vi "子vi调用.vi"() -> ()   [LabVIEW 2018]
panel:
  in  "布尔":bool
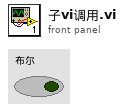
[diagram p1: front panel]
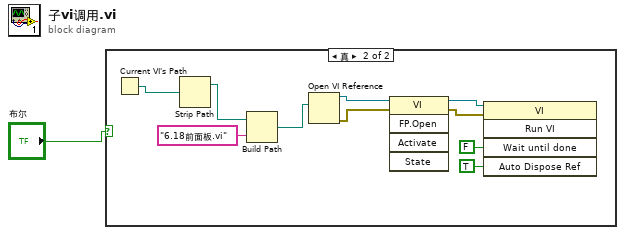
[diagram p0: block diagram]
diagram:
  n1 = case shown="真" "布尔" {
    frame False {
    }
    frame True {
      n2 = Current VI's Path() -> (path=w11:path)
      n3 = Strip Path(path=w11) -> (stripped path=w10:path)  [unwired: 1 out]
      n4 = Build Path(base path=w10, name or relative path="6.18前面板.vi" ("名称或相对路径")) -> (appended path=w8:path)
      n5 = Open VI Reference(vi path=w8) -> (vi reference=w7:refnum<vi>, error out=w6:errorcluster)  [unwired: 5 in]
      n6 = invoke class="VI" method="FP.Open"(reference=w7, error in=w6) -> (reference out=w5:refnum<vi>, error out=w4:errorcluster)  [unwired: 3 in, 3 out]
      n7 = invoke class="VI" method="Run VI"(reference=w5, error in=w4, "Wait until done"=FALSE ("结束前等待"), "Auto Dispose Ref"=TRUE ("自动销毁引用")) -> ()  [unwired: 1 in, 5 out]
    }
  }
